vi "Main.vi"() -> ()   [LabVIEW 2015, in "User 2.lvlib"]
doc: "This template is based off of the Queued Message Handler design pattern and the Queued Message Handler project template that ships with LabVIEW.\n\nThe main difference is that the queue is private to this module and communication between modules is performed via Broadcast and Request events.\n\nRequest events are wrapped in public API methods and are handled in the Event Handling Loop (EHL) of this VI. Any module can register for Broadcast events sent by this module. The EHL generates messages based on user interface actions.\n\nThe Message Handling Loop (MHL) processes messages generated by the EHL, or by other messages. The messages are string values, so new messages can be added easily to the Message Cases case structure in the MHL. Each message cluster can also provide an optional value for Message Data, which is a variant that can be converted to whatever message-specific data is required.\n_____\nBased on Delacor QMH Project Template 4.2.1.64."
uses:
  User 2.lvlib
  <vilib>/Delacor/Delacor QMH/Libraries/Module Admin_class/Delacor_lib_QMH_Module Admin.lvclass
  Module Data--cluster.ctl
  <vilib>/Delacor/Delacor QMH/Libraries/Message Queue_class/Delacor_lib_QMH_Message Queue.lvclass/Delacor_lib_QMH_Message Queue.ctl
  Stop Argument--cluster.ctl
  <vilib>/Delacor/Delacor QMH/Libraries/Module Admin_class/Delacor_lib_QMH_Module Admin.lvclass/Delacor_lib_QMH_Module Admin.ctl
  Update screen Argument--cluster.ctl
  <vilib>/Utility/miscctls.llb/LVPointTypeDef.ctl
  <vilib>/Delacor/Delacor QMH/Libraries/Message Queue_class/Delacor_lib_QMH_Enqueue Message (Single).vi
  <vilib>/Delacor/Delacor QMH/Libraries/Module Admin_class/Delacor_lib_QMH_Get External Launch.vi
  <vilib>/Utility/error.llb/Error Cluster From Error Code.vi
  <vilib>/ErrorRing/Error Ring.xnode
  <vilib>/Delacor/Delacor QMH/Libraries/Message Queue_class/Delacor_lib_QMH_Message Queue.lvclass
panel:
  in  "Send!":bool
  out "Message":string
  in  "Message to send":string
  in  "Simulate MHL Error":bool
  in  "Simulate EHL Error":bool
  out "error out":errorcluster
  in  "Module Admin":refnum<class "Delacor_lib_QMH_Module Admin.lvclass">
  out "Status":string
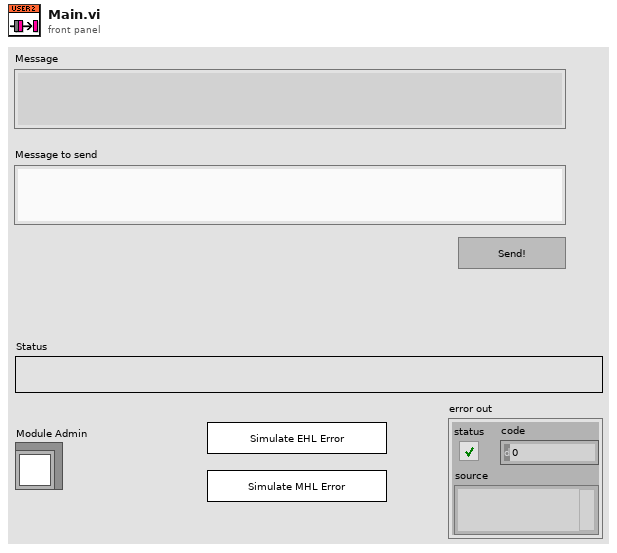
[diagram p1: front panel]
types:
  T1 = typedef "User 2.lvlib/Request Events--cluster.ctl" = cluster{"Stop Module":refnum<user-event>, "Show Panel":refnum<user-event>, "Hide Panel":refnum<user-event>, "Get Module Execution Status":refnum<user-event>, "Show Diagram":refnum<user-event>, "Update screen":refnum<user-event>}
  T2 = typedef "User 2.lvlib/Module Data--cluster.ctl" = cluster{"Status":string}
  T3 = enum32{"invalid lock state", "Not Locked", "Locked (No Password)", "Password-protected"}
  T4 = typedef "User 2.lvlib/Stop Argument--cluster.ctl" = cluster{"Origin":string, "Exit via Stop Module Req?":bool, "Wait for Module to stop?":bool}
  T5 = typedef "User 2.lvlib/Update screen Argument--cluster.ctl" = cluster{"Message":string}
  T6 = typedef "LVPointTypeDef.ctl" = cluster{"Horizontal":i16, "Vertical":i16}
  T7 = enum32{"Invalid", "Standard", "Closed", "Hidden", "Minimized", "Maximized"}
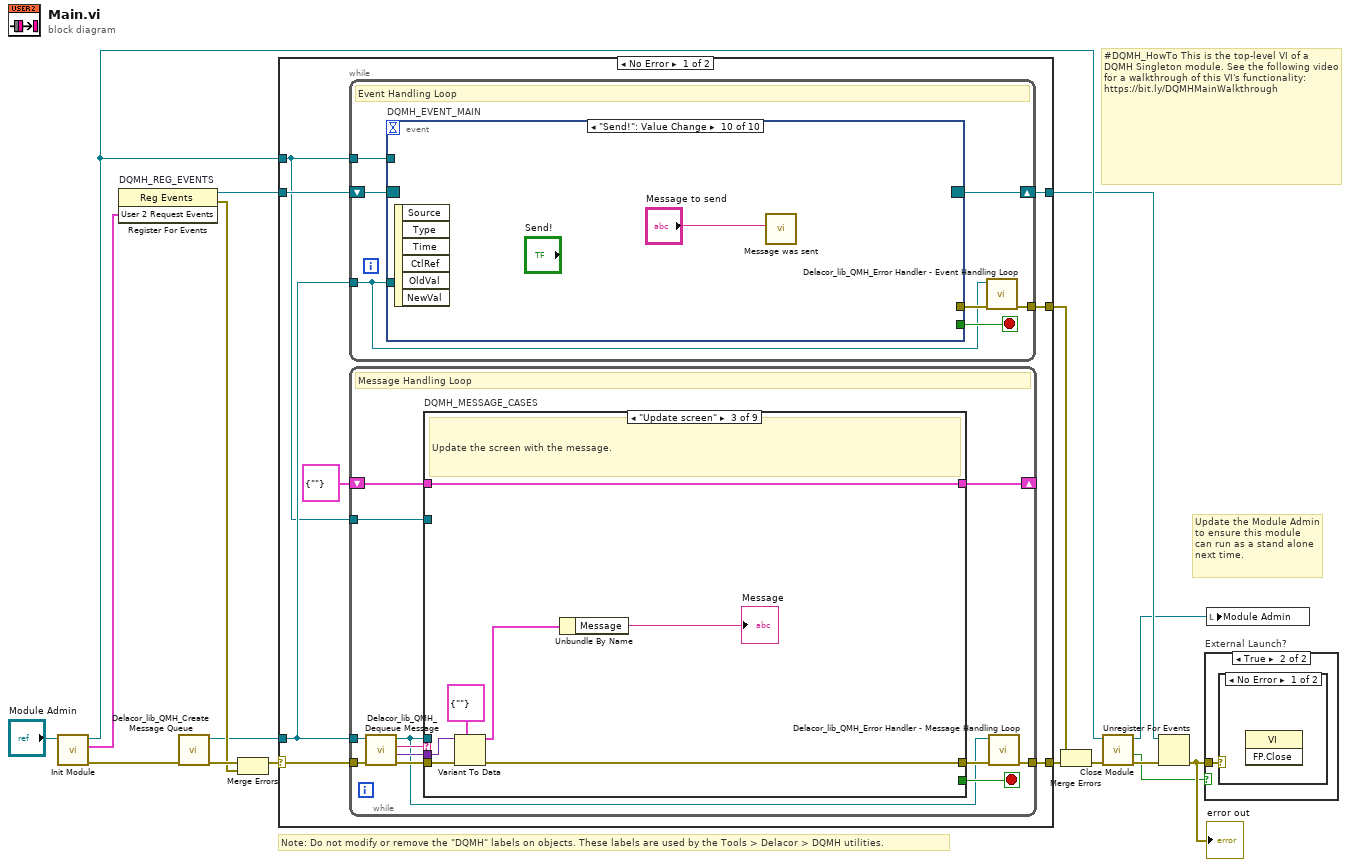
[diagram p0: block diagram]
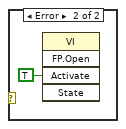
[diagram p3: hidden frame]
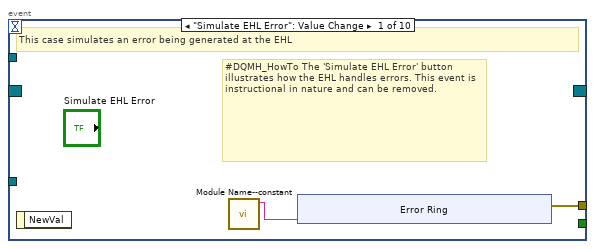
[diagram p4: hidden frame]
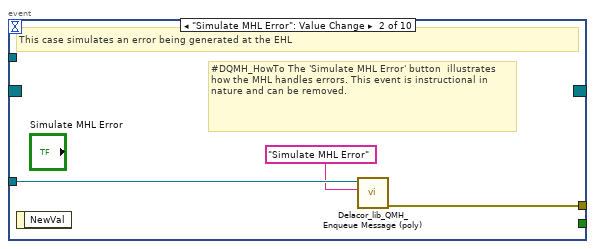
[diagram p5: hidden frame]
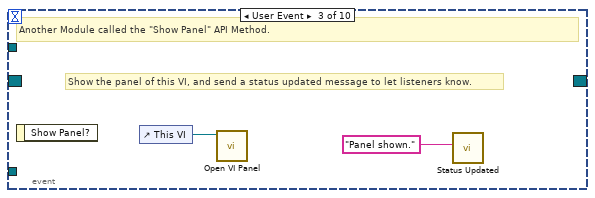
[diagram p6: hidden frame]
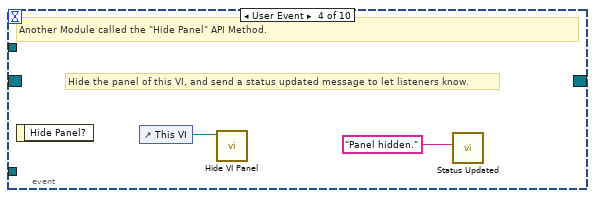
[diagram p7: hidden frame]
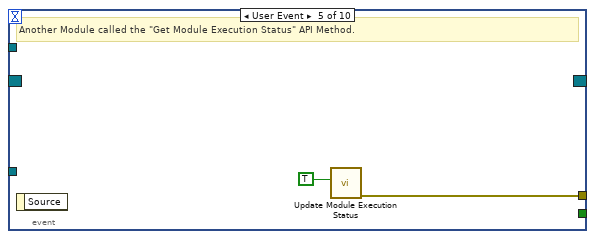
[diagram p8: hidden frame]
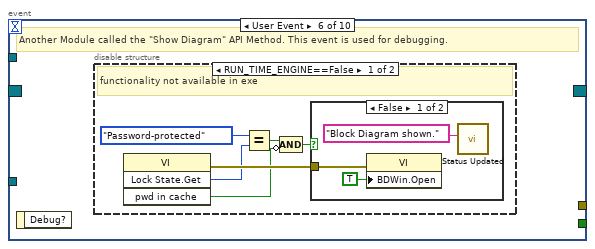
[diagram p9: hidden frame]
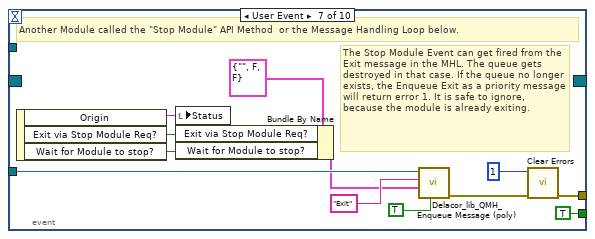
[diagram p12: hidden frame]
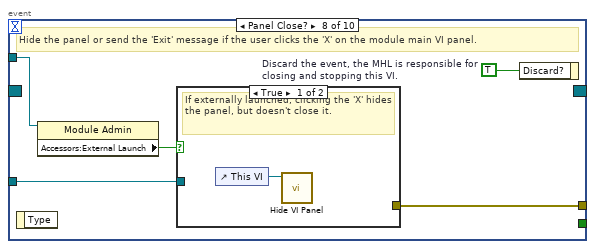
[diagram p13: hidden frame]
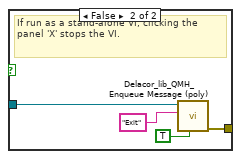
[diagram p14: hidden frame]
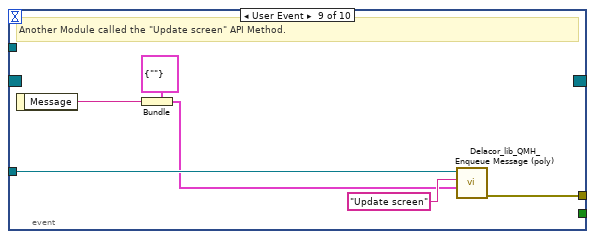
[diagram p15: hidden frame]
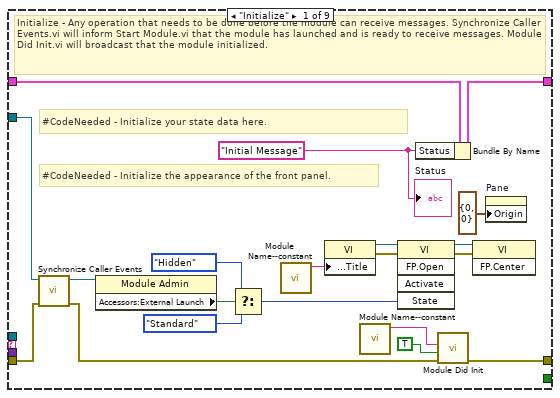
[diagram p16: hidden frame]
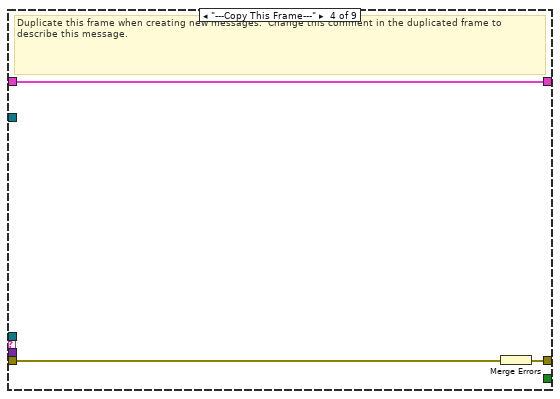
[diagram p18: hidden frame]
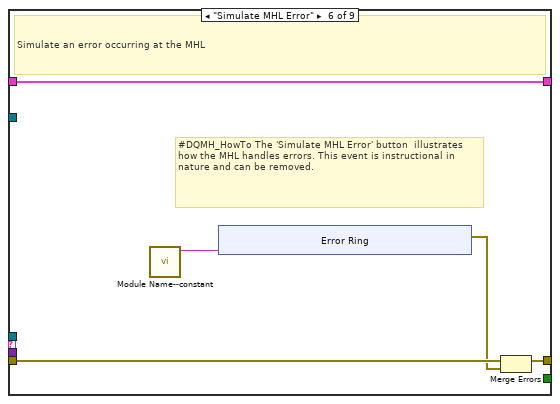
[diagram p20: hidden frame]
diagram:
  # "#DQMH_HowTo This is the top-level VI of a DQMH Singleton module. See the following video for a walkthrough of this VI's functionality: https://bit.ly/DQMHMainWalkthrough"
  # "Note: Do not modify or remove the \"DQMH\" labels on objects. These labels are used by the Tools > Delacor > DQMH utilities."
  # "Update the Module Admin to ensure this module can run as a stand alone next time."
  n1 = call "Init Module.vi"("Singleton Module Admin in"="Module Admin") -> ("error out"=w16:errorcluster, "User 2 Request Events"=w5:T1, "Singleton Module Admin out"=w8:refnum<class "Delacor_lib_QMH_Module Admin.lvclass">)  [unwired: 8 in]
  n2 = register-events "DQMH_REG_EVENTS"(w5) -> (reference out=w6:refnum<event-registration>, error out=w9:errorcluster)  [unwired: 2 in]
  n3 = call <vilib>:"Delacor_lib_QMH_Create Message Queue.vi"("error in (no error)"=w16) -> ("error out"=w11:errorcluster, "Message Queue"=w4:refnum<class "Delacor_lib_QMH_Message Queue.lvclass">)  [unwired: 9 in]
  n4 = Merge Errors(w11, w9) -> (w10:errorcluster)
  n5 = case shown="No Error" w10 {
    selector: w10 -> [w23 w199]
    tunnel: [w25 w199] -> w17
    tunnel: [w22 w196] -> w7
    tunnel: w6 -> [w20 w196]
    tunnel: w4 -> [w19 _]
    tunnel: [w24 _] -> w14
    tunnel: w8 -> [w18 w192]
    frame No Error {
      n6 = while {
        tunnel: w19 -> [w26]
        shift-right: [w29] -> w22
        shift-left: w20 -> [w30]
        tunnel: [w31] -> w24
        tunnel: w18 -> [w27]
        stop <- w28 stop-if-true
        # "Event Handling Loop"
        n7 = event "DQMH_EVENT_MAIN" shown="[9] \"Send!\": Value Change" {
          selector: w30 -> [_ _ _ _ _ _ _ _ _ _]
          dyn-events: [_ _ _ _ _ _ _ _ _ _] -> w29
          timeout: _ -> [_ _ _ _ _ _ _ _ _ _]
          tunnel: [_ _ _ _ _ _ TRUE ("Discard?") _ _ _] -> w28
          tunnel: w26 -> [_ w43 _ _ _ _ w67 w74 w87 _]
          tunnel: [w34 w44 _ _ w50 _ w70 w76 w83 _] -> w32
          tunnel: w27 -> [_ _ _ _ _ _ _ w73 _ _]
          event "Simulate EHL Error": Value Change {
            # "#DQMH_HowTo The 'Simulate EHL Error' button  illustrates how the EHL handles errors. This event is instructional in nature and can be removed."
            # "This case simulates an error being generated at the EHL"
            n8 = event-data() -> ()  [unwired: 1 in, 1 out]
            n9 = call "Module Name--constant.vi"() -> ("Module Name"=w33:string)  [unwired: 11 in]
            n10 = xnode "Error Ring"("parameter 0"=w33) -> ("error out"=w34:errorcluster)
          }
          event "Simulate MHL Error": Value Change {
            # "#DQMH_HowTo The 'Simulate MHL Error' button  illustrates how the MHL handles errors. This event is instructional in nature and can be removed."
            # "This case simulates an error being generated at the EHL"
            n11 = event-data() -> ()  [unwired: 1 in, 1 out]
            n12 = call-poly <vilib>:"Delacor_lib_QMH_Enqueue Message (poly).vi"("Message"="Simulate MHL Error", "Message Queue in"=w43) -> ("error out"=w44:errorcluster)  [unwired: 8 in, 1 out]
          }
          event User Event {
            # "Show the panel of this VI, and send a status updated message to let listeners know."
            # "Another Module called the \"Show Panel\" API Method."
            n13 = event-data() -> ()  [unwired: 1 in, 1 out]
            n14 = control-ref of="This VI"() -> (w46:refnum<vi>)
            n15 = call "Open VI Panel.vi"("VI"=w46) -> ()  [unwired: 10 in, 1 out]
            n16 = call "Status Updated.vi"("Status"="Panel shown." ("format string")) -> ()  [unwired: 10 in, 1 out]
          }
          event User Event {
            # "Hide the panel of this VI, and send a status updated message to let listeners know."
            # "Another Module called the \"Hide Panel\" API Method."
            n17 = event-data() -> ()  [unwired: 1 in, 1 out]
            n18 = control-ref of="This VI"() -> (w48:refnum<vi>)
            n19 = call "Hide VI Panel.vi"("VI"=w48) -> ()  [unwired: 10 in, 1 out]
            n20 = call "Status Updated.vi"("Status"="Panel hidden." ("format string")) -> ()  [unwired: 10 in, 1 out]
          }
          event User Event {
            # "Another Module called the \"Get Module Execution Status\" API Method."
            n21 = event-data() -> ()  [unwired: 1 in, 1 out]
            n22 = call "Update Module Execution Status.vi"("Running?"=TRUE) -> ("error out"=w50:errorcluster)  [unwired: 10 in]
          }
          event User Event {
            # "Another Module called the \"Show Diagram\" API Method. This event is used for debugging."
            n23 = event-data() -> ()  [unwired: 1 in, 1 out]
            n24 = disable-structure shown="RUN_TIME_ENGINE==False" {
              frame condition #0 (active) {
                # "functionality not available in exe"
                n25 = invoke class="VI" method="Lock State.Get"() -> (error out=w56:errorcluster, "Get Lock State"=w55:T3, "pwd in cache"=w52:bool)  [unwired: 4 in, 1 out]
                n26 = Equal?(x=T3."Password-protected", y=w55) -> (x = y?=w53:bool)
                n27 = Compound Arithmetic op=AND(w53, invert w52) -> (w51:bool)
                n28 = case shown="False" w51 {
                  tunnel: w56 -> [w59 _]
                  frame False {
                    n29 = property class="VI"(error in=w59, "BDWin.Open"=TRUE ("Block Diagram Window:Open")) -> ()  [unwired: 1 in, 2 out]
                    n30 = call "Status Updated.vi"("Status"="Block Diagram shown." ("format string")) -> ()  [unwired: 10 in, 1 out]
                  }
                  frame True {
                    # "Password-protected VI, and the password is not in the cache. Do not show the diagram."
                  }
                }
              }
              frame condition #1 {
              }
            }
          }
          event User Event {
            # "The Stop Module Event can get fired from the Exit message in the MHL. The queue gets destroyed in that case. If the queue no longer exists, the Enqueue Exit as a priority message will return error 1. It is safe to ignore, because the module is already exiting."
            # "Another Module called the \"Stop Module\" API Method  or the Message Handling Loop below."
            n31 = event-data() -> ("Origin"=w66:string, "Exit via Stop Module Req?"=w62:bool, "Wait for Module to stop?"=w61:bool)  [unwired: 1 in]
            n32 = local write "Status"(w66) -> ()
            n33 = Bundle By Name(cluster=T4 {"Origin"="", "Exit via Stop Module Req?"=FALSE, "Wait for Module to stop?"=FALSE} ("Stop Argument"), "Exit via Stop Module Req?"=w62, "Wait for Module to stop?"=w61) -> (w60:T4)
            n34 = call-poly <vilib>:"Delacor_lib_QMH_Enqueue Message (poly).vi"("Priority Message? (F)"=TRUE, "Message Data"=w60, "Message"="Exit", "Message Queue in"=w67) -> ("error out"=w71:errorcluster)  [unwired: 6 in, 1 out]
            n35 = call <vilib>:"Clear Errors.vi"("error in (no error)"=w71, "specific error code to clear (0: all)"=1) -> ("error out"=w70:errorcluster)  [unwired: 4 in, 1 out]
          }
          event Panel Close? {
            w75 = TRUE  # Discard the event, the MHL is responsible for closing and stopping this VI.
            # "Hide the panel or send the 'Exit' message if the user clicks the 'X' on the module main VI panel."
            n36 = event-data() -> ()  [unwired: 1 in, 1 out]
            n37 = property class="Module Admin"(reference=w73) -> ("Accessors:External Launch"=w72:bool)  [unwired: 1 in, 2 out]
            n38 = case shown="True" w72 {
              tunnel: w74 -> [_ w80]
              tunnel: [_ w81] -> w76
              frame True {
                # "If externally launched, clicking the 'X' hides the panel, but doesn't close it."
                n39 = control-ref of="This VI"() -> (w77:refnum<vi>)
                n40 = call "Hide VI Panel.vi"("VI"=w77) -> ()  [unwired: 10 in, 1 out]
              }
              frame False {
                # "If run as a stand-alone VI, clicking the panel 'X' stops the VI."
                n41 = call-poly <vilib>:"Delacor_lib_QMH_Enqueue Message (poly).vi"("Priority Message? (F)"=TRUE, "Message"="Exit", "Message Queue in"=w80) -> ("error out"=w81:errorcluster)  [unwired: 7 in, 1 out]
              }
            }
            n42 = event-data("Discard?"=w75) -> ()  [unwired: 1 in, 1 out]
          }
          event User Event {
            # "Another Module called the \"Update screen\" API Method."
            n43 = event-data() -> ("Message"=w82:string)  [unwired: 1 in]
            n44 = Bundle(cluster=T5 {"Message"=""} ("Update screen Argument"), "Message"=w82) -> (w84:T5)
            n45 = call-poly <vilib>:"Delacor_lib_QMH_Enqueue Message (poly).vi"("Message Data"=w84, "Message"="Update screen", "Message Queue in"=w87) -> ("error out"=w83:errorcluster)  [unwired: 7 in, 1 out]
          }
          event "Send!": Value Change {
            n46 = event-data() -> ()  [unwired: 1 in, 6 out]
            n47 = call "Message was sent.vi"("Message"="Message to send") -> ()  [unwired: 10 in, 1 out]
          }
        }
        n48 = call-dynamic "Delacor_lib_QMH_Error Handler - Event Handling Loop.vi"("error in (no error)"=w32, "Message Queue in"=w26) -> ("dup error in"=w31:errorcluster)  [unwired: 8 in, 1 out]
      }
      n49 = while {
        tunnel: w19 -> [w91]
        shift-right: [w95] -> _
        shift-left: T2 {"Status"=""} ("Data Cluster") -> [w96]
        tunnel: w23 -> [w99]
        tunnel: [w97] -> w25
        tunnel: w18 -> [w89]
        stop <- w94 stop-if-true
        # "Message Handling Loop"
        n50 = call-dynamic "Delacor_lib_QMH_Dequeue Message.vi"("error in (no error)"=w99, "Message Queue in"=w91) -> ("error out"=w98:errorcluster, "Message Data"=w92:variant, "Message"=w93:string, "Message Queue out"=w90:refnum<class "Delacor_lib_QMH_Message Queue.lvclass">)  [unwired: 6 in]
        n51 = case "DQMH_MESSAGE_CASES" shown="\"Update screen\"" w93 {
          selector: w93 -> [_ _ _ _ _ _ _ _ w179]
          tunnel: w90 -> [_ _ _ _ _ _ w149 w171 _]
          tunnel: w98 -> [w118 w122 w129 w132 w134 w139 w156 w177 w181]
          tunnel: [w116 w122 w127 w131 w134 w138 w152 w174 w182] -> w100
          tunnel: w96 -> [w107 w121 w128 w130 w133 w136 w151 w170 w180]
          tunnel: [w106 w121 w128 w130 w133 w136 w151 w170 w180] -> w95
          tunnel: [_ _ _ _ _ _ _ w169 _] -> w94
          tunnel: w92 -> [_ _ w126 _ _ _ w150 w168 _]
          tunnel: w89 -> [w108 _ _ _ _ _ w148 w163 _]
          frame "Initialize" {
            w101 = "Initial Message" ("Initial Message")
            # "#CodeNeeded - Initialize the appearance of the front panel."
            # "#CodeNeeded - Initialize your state data here."
            # "Initialize - Any operation that needs to be done before the module can receive messages. Synchronize Caller Events.vi will inform Start Module.vi that the module has launched and is ready to receive messages. Module Did Init.vi will broadcast that the module initialized."
            n52 = call "Synchronize Caller Events.vi"("error in (no error)"=w118, "Singleton Module Admin in"=w108) -> ("error out"=w117:errorcluster, "Singleton Module Admin out"=w103:refnum<class "Delacor_lib_QMH_Module Admin.lvclass">)  [unwired: 8 in]
            n53 = property class="Module Admin"(reference=w103) -> ("Accessors:External Launch"=w112:bool)  [unwired: 1 in, 2 out]
            n54 = Select(t=T7."Hidden" ("State"), s=w112, f=T7."Standard" ("State")) -> (s? t:f=w109:T7)
            n55 = call "Module Name--constant.vi"() -> ("Module Name"=w115:string)  [unwired: 11 in]
            n56 = property class="VI"("Front Panel.Title"=w115) -> (reference out=w114:refnum<vi>, error out=w120:errorcluster)  [unwired: 2 in]
            n57 = call "Module Name--constant.vi"() -> ("Module Name"=w104:string)  [unwired: 11 in]
            n58 = invoke class="VI" method="FP.Open"(reference=w114, error in=w120, "State"=w109) -> (reference out=w113:refnum<vi>, error out=w119:errorcluster)  [unwired: 2 in, 3 out]
            n59 = Bundle By Name(cluster=w107, "Status"=w101) -> (w106:T2)
            n60 = call "Module Did Init.vi"("error in (no error)"=w117, "Initialized?"=TRUE, "Origin"=w104) -> ("error out"=w116:errorcluster)  [unwired: 8 in]
            n61 = invoke class="VI" method="FP.Center"(reference=w113, error in=w119) -> ()  [unwired: 1 in, 3 out]
            n62 = property on="Pane" class="Pane"("Origin"=T6 {"Horizontal"=0, "Vertical"=0}) -> ()  [unwired: 2 in, 2 out]
            "Status" <- w101
          }
          frame "--- Module Specific ---" {
            # "Separator -- The following cases handle messages specific to this Module."
          }
          frame "Update screen" {
            # "Update the screen with the message."
            n63 = Variant To Data(error in=w129, type=T5 {"Message"=""} ("Update screen Argument"), Variant=w126) -> (data=w124:T5, error out=w127:errorcluster)
            n64 = Unbundle By Name(w124) -> ("Message"=→"Message":string)
          }
          frame "---Copy This Frame---" {
            # "Duplicate this frame when creating new messages.  Change this comment in the duplicated frame to describe this message."
            n65 = Merge Errors(w132) -> (w131:errorcluster)
          }
          frame "--- Exit and Error Handling---" {
            # "Separator - The following cases handle errors and exit messages."
          }
          frame "Simulate MHL Error" {
            # "#DQMH_HowTo The 'Simulate MHL Error' button  illustrates how the MHL handles errors. This event is instructional in nature and can be removed."
            # "Simulate an error occurring at the MHL"
            n66 = call "Module Name--constant.vi"() -> ("Module Name"=w135:string)  [unwired: 11 in]
            n67 = xnode "Error Ring"("parameter 0"=w135) -> ("error out"=w137:errorcluster)
            n68 = Merge Errors(w139, w137) -> (w138:errorcluster)
          }
          frame "Error" {
            # "#CodeRecommended - If you ever change the name of this \"Error\" message, you'll need to update the name in the Check Loop Error.vi as well."
            # "#CodeRecommended - If the module is running in standalone mode (External Launch = FALSE), this code will pop up an error dialog and call the 'Exit' message if an error occurs. Add more fine-grained error handling here."
            # "Error - Check the error message data and respond accordingly. This message is sent by the \"Error Handler\" VIs at the end of each loop in this application."
            n69 = property class="Module Admin"(reference=w148) -> ("Accessors:External Launch"=w147:bool)  [unwired: 1 in, 2 out]
            n70 = Variant To Data(error in=w156, type=errorcluster {"status"=FALSE, "code"=0, "source"=""} ("error constant"), Variant=w150) -> (data=w157:errorcluster, error out=w154:errorcluster)
            n71 = call "Error Reported.vi"("Error"=w157) -> ()  [unwired: 10 in, 1 out]
            n72 = case shown="False" w147 {
              tunnel: [w162 _] -> w153
              tunnel: w149 -> [w160 _]
              tunnel: w157 -> [w161 _]
              frame False {
                # "If the module is running standalone, then pop up an error dialog and call the \"Exit\" message."
                n73 = call <vilib>:"Simple Error Handler.vi"("error in (no error)"=w161) -> ()  [unwired: 4 in, 5 out]
                n74 = call-poly <vilib>:"Delacor_lib_QMH_Enqueue Message (poly).vi"("Priority Message? (F)"=TRUE, "Message"="Exit", "Message Queue in"=w160) -> ("error out"=w162:errorcluster)  [unwired: 7 in, 1 out]
              }
              frame True {
                # "If the module was launched externally, calling the Error Reported broadcast VI is the only action performed by the \"Error\" message. The module's caller can then process the error appropriately."
              }
            }
            n75 = Merge Errors(w154, w153) -> (w152:errorcluster)
            n76 = local write "error out"(w152) -> ()
          }
          frame "Exit" {
            w167 = 91  # 91: not all Exit messages will have an argument
            w169 = TRUE  # Stop the VI
            # "Release the message queue reference"
            # "#CodeNeeded - Add any required cleanup code here"
            # "Exit - Exit the application."
            n77 = Variant To Data(error in=w177, type=T4 {"Origin"="", "Exit via Stop Module Req?"=FALSE, "Wait for Module to stop?"=FALSE} ("Stop Argument"), Variant=w168) -> (data=w165:T4, error out=w173:errorcluster)
            n78 = call <vilib>:"Clear Errors.vi"("error in (no error)"=w173, "specific error code to clear (0: all)"=w167) -> ("error out"=w176:errorcluster)  [unwired: 4 in, 1 out]
            n79 = control-ref of="This VI"() -> (w164:refnum<vi>)
            n80 = call-dynamic "Delacor_lib_QMH_Release Message Queue.vi"("error in (no error)"=w176, "Message Queue"=w171) -> ("error out"=w175:errorcluster)  [unwired: 9 in]
            n81 = call "Handle Exit.vi"("Stop Argument"=w165, "Admin in"=w163, "VI reference"=w164) -> ("error out"=w172:errorcluster)  [unwired: 7 in, 1 out]
            n82 = Merge Errors(w175, w172) -> (w174:errorcluster)
          }
          frame Default {
            # "'Default' case only runs if there is a message that isn't defined in any of the other cases.  Output a programming error."
            n83 = call "Module Name--constant.vi"() -> ("Module Name"=w178:string)  [unwired: 11 in]
            n84 = xnode "Error Ring"("parameter 0"=w179, "parameter 1"=w178) -> ("error out"=w183:errorcluster)
            n85 = Merge Errors(w181, w183) -> (w182:errorcluster)
          }
        }
        n86 = call-dynamic "Delacor_lib_QMH_Error Handler - Message Handling Loop.vi"("error in (no error)"=w100, "Message Queue in"=w90) -> ("dup error in"=w97:errorcluster)  [unwired: 8 in, 1 out]
      }
    }
    frame Error {
      # "Synchronize Caller Events.vi will inform Start Module.vi that the module has launched and will let the code calling Start Module.vi register for broadcasts and would permit the caller receive the broadcast that an error occurred at launch time."
      n87 = call "Synchronize Caller Events.vi"("Singleton Module Admin in"=w192) -> ("error out"=w197:errorcluster)  [unwired: 9 in, 1 out]
      n88 = call "Module Name--constant.vi"() -> ("Module Name"=w195:string)  [unwired: 11 in]
      n89 = Format Into String(format string="An error occurred during initialization. %s is no longer running.", w195) -> (resulting string=w193:string)  [unwired: 2 in, 1 out]
      n90 = Merge Errors(w199, w197) -> (w198:errorcluster)
      n91 = call "Error Reported.vi"("Additional Information"=w193, "Error"=w198) -> ()  [unwired: 9 in, 1 out]
    }
  }
  n92 = Merge Errors(w14, w17) -> (w13:errorcluster)
  n93 = call "Close Module.vi"("error in (no error)"=w13, "Module Admin in"=w8) -> ("error out"=w15:errorcluster, "External Launch"=w1:bool, "Module Admin out"=w2:refnum<class "Delacor_lib_QMH_Module Admin.lvclass">)  [unwired: 7 in]
  n94 = Unregister For Events(event registration refnum=w7, error in=w15) -> (error out=w12:errorcluster)
  "error out" <- w12
  n95 = case "External Launch?" shown="True" w1 {
    tunnel: w12 -> [_ w200]
    frame False {
    }
    frame True {
      n96 = case shown="No Error" w200 {
        frame No Error {
          n97 = invoke class="VI" method="FP.Close"() -> ()  [unwired: 3 in, 3 out]
        }
        frame Error {
          n98 = invoke class="VI" method="FP.Open"("Activate"=TRUE ("Activate?")) -> ()  [unwired: 4 in, 5 out]
        }
      }
    }
  }
  n99 = local write "Module Admin"(w2) -> ()
